vi "CreateFrontPanelImage.vi"(8 "error (in)":errorcluster, 10 "VI Path":path, 11 "VI in":refnum<vi>) -> (0 "error (out)":errorcluster, 2 "Image Path":path, 3 "Panel out":refnum<vi>)   [LabVIEW 2017]
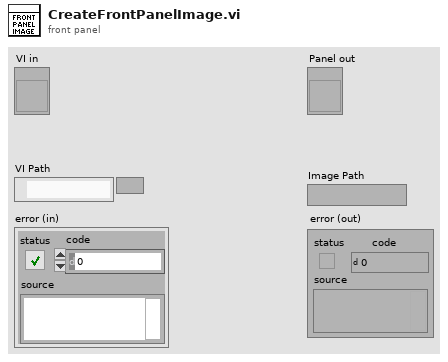
[diagram p1: front panel]
types:
  T1 = typedef "imagedata.ctl" = cluster{"image type":i32, "image depth":i32, "image":u8[], "mask":u8[], "colors":u32[], "Rectangle":cluster{"left":i16, "top":i16, "right":i16, "bottom":i16}}
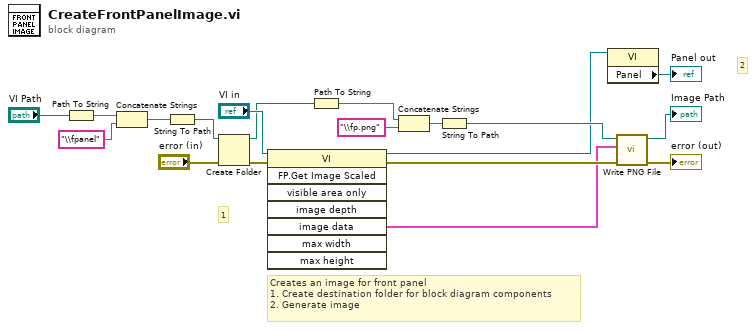
[diagram p0: block diagram]
diagram:
  # "2"
  # "1"
  # "Creates an image for front panel\n1. Create destination folder for block diagram components\n2. Generate image"
  n1 = Path To String(path="VI Path") -> (string=w17:string)
  n2 = Concatenate Strings(w17, "\\fpanel" ("string")) -> (w15:string)
  n3 = String To Path(string=w15) -> (path=w14:path)
  n4 = Create Folder(path (use dialog)=w14, error in="error (in)") -> (created path=w11:path, error out=w12:errorcluster)  [unwired: 1 in, 1 out]
  n5 = invoke class="VI" method="FP.Get Image Scaled"(reference="VI in", error in=w12) -> (reference out=w2:refnum<vi>, error out=w6:errorcluster, "image data"=w3:T1)  [unwired: 6 in, 5 out]
  n6 = Path To String(path=w11) -> (string=w10:string)
  n7 = Concatenate Strings(w10, "\\fp.png" ("string")) -> (w8:string)
  n8 = String To Path(string=w8) -> (path=w7:path)
  n9 = property class="VI"(reference=w2) -> ("Panel"=→"Panel out":refnum<vi>)  [unwired: 1 in, 2 out]
  n10 = call <vilib>:"Write PNG File.vi"("error in (no error)"=w6, "image data"=w3, "path to PNG file"=w7) -> ("error out"=→"error (out)":errorcluster, "path"=→"Image Path":path)  [unwired: 7 in]
